vi "Test Overflow 2.vi"() -> ()   [LabVIEW 2014, in "Arduino SoftwareSerial Wrapper.lvlib"]
uses:
  Arduino SoftwareSerial Wrapper.lvlib
panel:
  out "Overflow?":bool
  out "Error Out":errorcluster
  in  "Error In":errorcluster
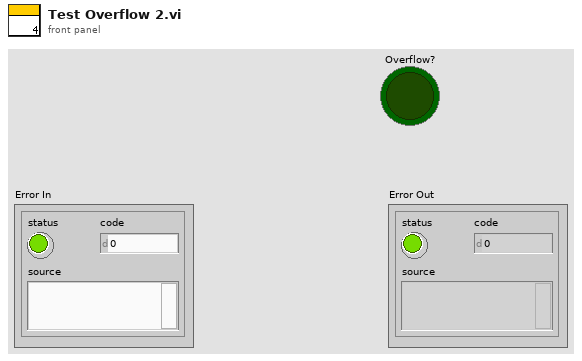
[diagram p1: front panel]
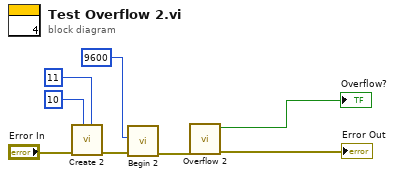
[diagram p0: block diagram]
diagram:
  n1 = call "Create 2.vi"("arduino RX pin"=u8 11 ("arduino TX pin"), "arduino TX pin"=u8 10 ("arduino RX pin"), "Error In"="Error In") -> ("Error Out"=w4:errorcluster)  [unwired: 8 in]
  n2 = call "Begin 2.vi"("Error In"=w4, "Baudrate"=u16 9600) -> ("Error Out"=w3:errorcluster)  [unwired: 8 in]
  n3 = call "Overflow 2.vi"("Error In"=w3) -> ("Error Out"=→"Error Out":errorcluster, "Overflow?"=→"Overflow?":bool)  [unwired: 9 in]
